vi "Transmission Ratio Calculator v2.vi"(10 "Ankle Angle":dbl) -> (2 "R_tau":dbl)   [LabVIEW 2018]
uses:
  Constants and System Parameters.ctl
panel:
  out "Constants and System Parameters":T1
  # "Input:"
  # "Output:"
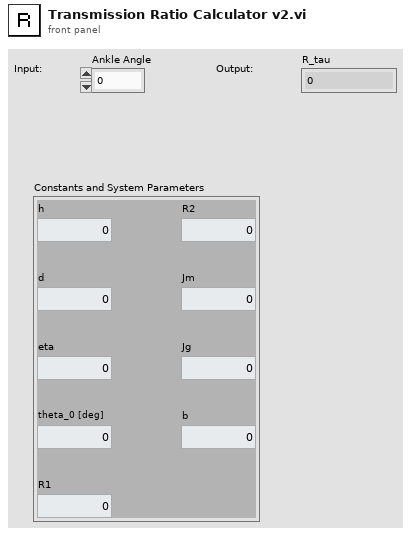
[diagram p1: front panel]
types:
  T1 = typedef "Constants and System Parameters.ctl" = cluster{"h":dbl, "d":dbl, "eta":dbl, "theta_0 [deg]":dbl, "R1":dbl, "R2":dbl, "Jm":dbl, "Jg":dbl, "b":dbl}
  T2 = cluster{"h":dbl, "d":dbl, "eta":dbl, "theta_0 [deg]":dbl, "R1":dbl, "R2":dbl, "Jm":dbl, "Jg":dbl, "b":dbl}
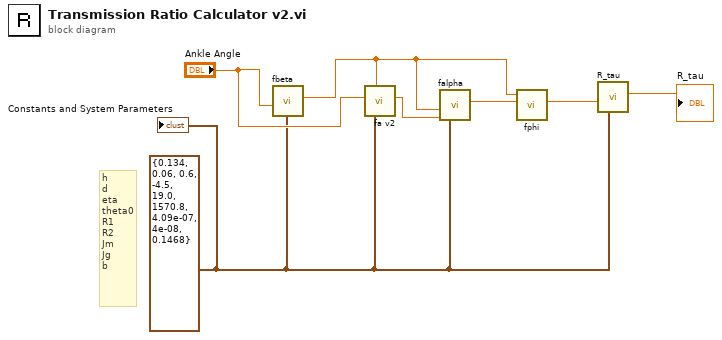
[diagram p0: block diagram]
diagram:
  w1 = T2 {"h"=0.134, "d"=0.06, "eta"=0.6, "theta_0 [deg]"=-4.5, "R1"=19.0, "R2"=1570.8, "Jm"=4.09e-07, "Jg"=4e-08, "b"=0.1468} ("Constants (system parameters)")
  # "h\nd\neta\ntheta0\nR1\nR2\nJm\nJg\nb"
  n1 = call "fbeta.vi"("Ankle Angle"="Ankle Angle", "Constants and System Parameters"=w1) -> ("fbeta"=w2:dbl)  [unwired: 9 in]
  n2 = call "fa v2.vi"("fbeta"=w2, "Constants and System Parameters"=w1, "Ankle Angle"="Ankle Angle") -> ("fa"=w3:dbl)  [unwired: 8 in]
  n3 = call "falpha.vi"("fa"=w3, "fbeta"=w2, "Constants and System Parameters"=w1) -> ("fapha"=w5:dbl)  [unwired: 8 in]
  n4 = call "fphi.vi"("fbeta"=w2, "falpha"=w5) -> ("fphi"=w6:dbl)  [unwired: 9 in]
  n5 = call "R_tau.vi"("fphi"=w6, "Constants and System Parameters"=w1) -> ("R_tau"=→"R_tau":dbl)  [unwired: 9 in]
  "Constants and System Parameters" <- w1
